vi "WPILogWaveformFromIndex.vi"(7 "XY Graph":refnum<vi>, 8 "error in (no error)":errorcluster, 9 "Index":i32, 10 "Graph Data":cluster{"X":dbl[], "Y":dbl[]}[](array[cluster]), 11 "Data Value Reference in":refnum<data-value>) -> (0 "error out":errorcluster, 2 "Graph Out":cluster{"X":dbl[], "Y":dbl[]}[](array[cluster]), 3 "Data Value Reference out":refnum<data-value>)   [LabVIEW 2020]
uses:
  Typedef/WPILibLog.ctl
  Typedef/Header.ctl
  Typedef/Entry.ctl
  Typedef/Record.ctl
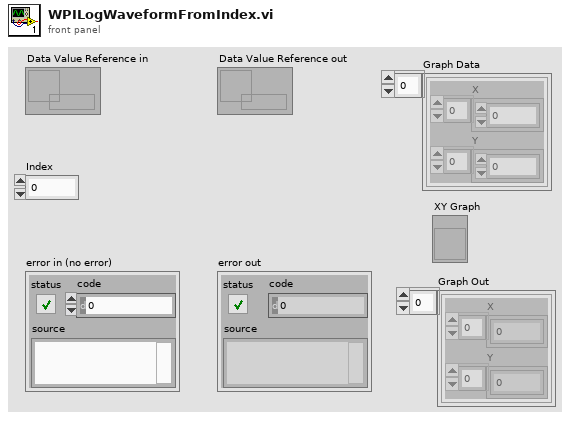
[diagram p1: front panel]
types:
  T1 = typedef "WPILibLog.ctl" = cluster{"Header":T2, "Record Start Idx":i32, "Entries":map{u32, T3}, "file ref":refnum<file>, "Finished Entries":T3[], "raw data":u8[]}
  T2 = typedef "Header.ctl" = cluster{"Header String":string, "Version":dbl, "Header Extra String Length":u32, "Header Extra String":string}
  T3 = typedef "Entry.ctl" = cluster{"ID":u32, "Records":T4[], "Finished?":bool, "Name":string, "Type":string, "Metadata":string, "RecordCnt":i32}
  T4 = typedef "Record.ctl" = cluster{"raw data":u8[], "ID":u32, "Size (bytes)":u32, "Timestamp":u64}
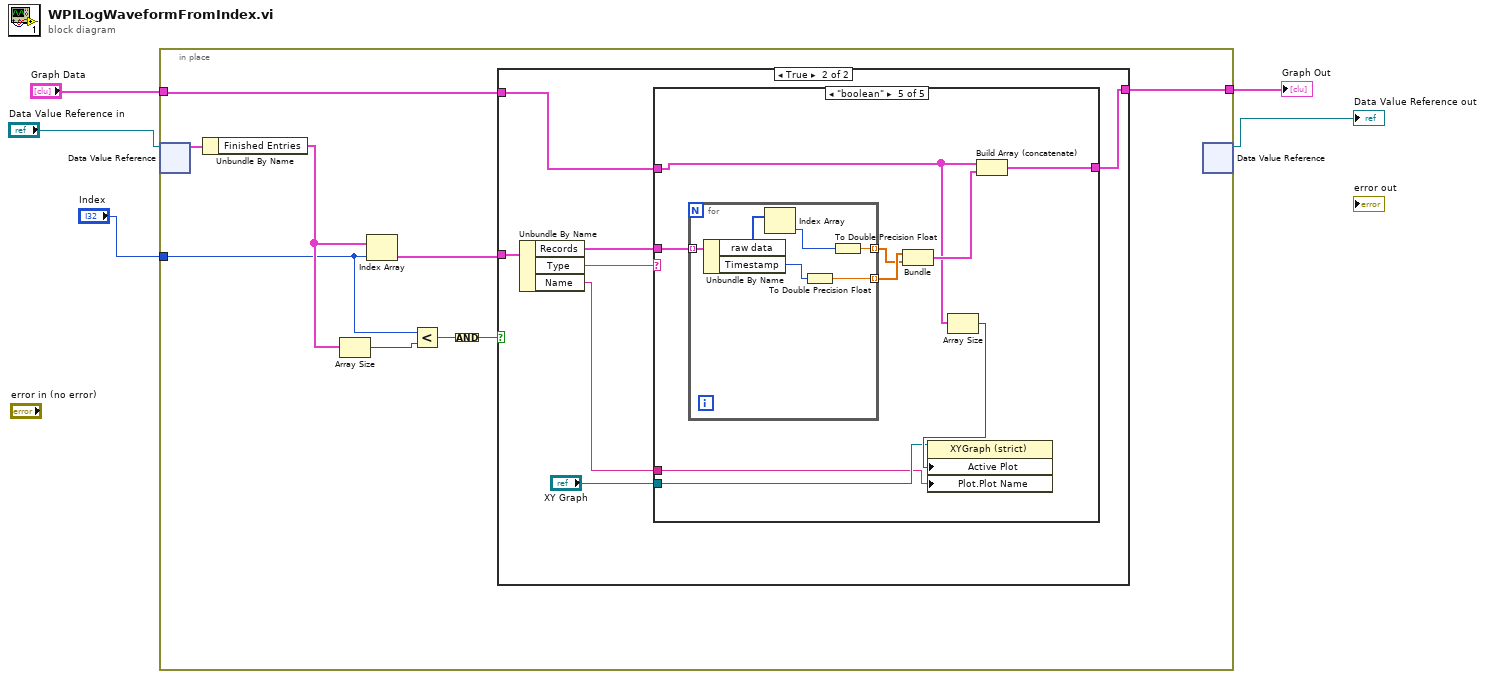
[diagram p0: block diagram]
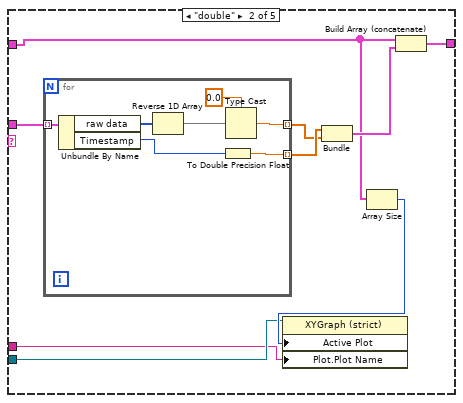
[diagram p4: hidden frame]
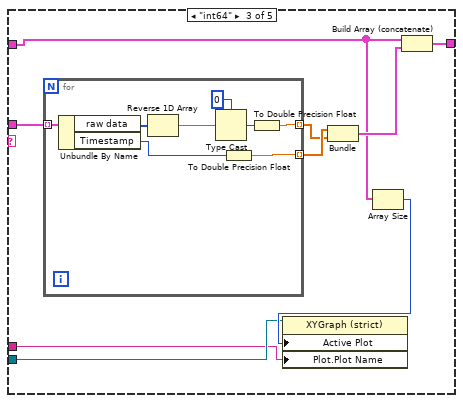
[diagram p5: hidden frame]
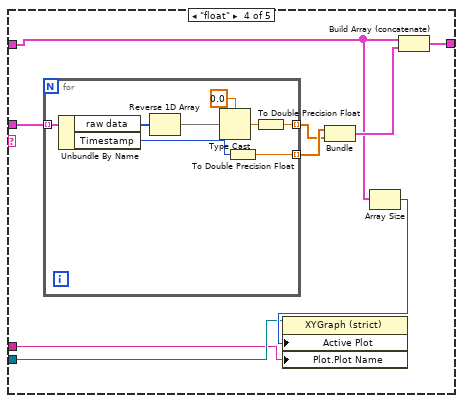
[diagram p6: hidden frame]
diagram:
  n1 = in-place {
    in-place-border: "Index" -> [w12]
    in-place-border: "Graph Data" -> [w7]
    in-place-border: [w6] -> w1
    n2 = in-place-dvr #1("Data Value Reference in") -> (w14:T1)  [unwired: 1 out]
    n3 = Unbundle By Name(w14) -> ("Finished Entries"=w13:T3[])
    n4 = Array Size(array=w13) -> (size(s)=w11:i32)
    n5 = Index Array(array=w13, index=w12) -> (element=w8:T3)
    n6 = Less?(x=w12, y=w11) -> (x < y?=w10:bool)
    n7 = Compound Arithmetic op=AND(w10) -> (w9:bool)
    n8 = case shown="True" w9 {
      tunnel: w8 -> [_ w22]
      tunnel: w7 -> [w15 w19]
      tunnel: [w15 w18] -> w6
      frame False {
      }
      frame True {
        n9 = Unbundle By Name(w22) -> ("Records"=w20:T4[], "Type"=w21:string, "Name"=w16:string)
        n10 = case shown="\"boolean\"" w21 {
          tunnel: w20 -> [_ w32 w48 w65 w82]
          tunnel: w19 -> [w23 w27 w43 w60 w77]
          tunnel: [w23 w28 w44 w61 w78] -> w18
          tunnel: "XY Graph" -> [_ w25 w41 w58 w75]
          tunnel: w16 -> [_ w24 w40 w57 w74]
          frame Default {
            # "Invalid Type, dont add"
          }
          frame "double" {
            n11 = for {
              tunnel: w32 -> [w39] mode=indexing
              tunnel: [w36] -> w30 mode=indexing
              tunnel: [w35] -> w31 mode=indexing
              n12 = Unbundle By Name(w39) -> ("raw data"=w38:u8[], "Timestamp"=w34:u64)
              n13 = Reverse 1D Array(array=w38) -> (reversed array=w33:u8[])
              n14 = To Double Precision Float(number=w34) -> (double precision float=w35:dbl)
              n15 = Type Cast(type=0.0, x=w33) -> (*(type *) &x=w36:dbl)
            }
            n16 = Bundle(w31, w30) -> (w29:cluster{dbl[], dbl[]})  [unwired: 1 in]
            n17 = Array Size(array=w27) -> (size(s)=w26:i32)
            n18 = property class="XYGraph (strict)"(reference=w25, "Active Plot"=w26, "Plot.Plot Name"=w24) -> ()  [unwired: 1 in, 2 out]
            n19 = Build Array (concatenate)(w27, w29) -> (w28:cluster{"X":dbl[], "Y":dbl[]}[])
          }
          frame "int64" {
            n20 = for {
              tunnel: w48 -> [w56] mode=indexing
              tunnel: [w51] -> w46 mode=indexing
              tunnel: [w52] -> w47 mode=indexing
              n21 = Unbundle By Name(w56) -> ("raw data"=w55:u8[], "Timestamp"=w50:u64)
              n22 = Reverse 1D Array(array=w55) -> (reversed array=w49:u8[])
              n23 = Type Cast(type=i64 0, x=w49) -> (*(type *) &x=w53:i64)
              n24 = To Double Precision Float(number=w50) -> (double precision float=w52:dbl)
              n25 = To Double Precision Float(number=w53) -> (double precision float=w51:dbl)
            }
            n26 = Bundle(w47, w46) -> (w45:cluster{dbl[], dbl[]})  [unwired: 1 in]
            n27 = Array Size(array=w43) -> (size(s)=w42:i32)
            n28 = property class="XYGraph (strict)"(reference=w41, "Active Plot"=w42, "Plot.Plot Name"=w40) -> ()  [unwired: 1 in, 2 out]
            n29 = Build Array (concatenate)(w43, w45) -> (w44:cluster{"X":dbl[], "Y":dbl[]}[])
          }
          frame "float" {
            n30 = for {
              tunnel: w65 -> [w73] mode=indexing
              tunnel: [w67] -> w63 mode=indexing
              tunnel: [w68] -> w64 mode=indexing
              n31 = Unbundle By Name(w73) -> ("raw data"=w72:u8[], "Timestamp"=w69:u64)
              n32 = Reverse 1D Array(array=w72) -> (reversed array=w66:u8[])
              n33 = Type Cast(type=sgl 0.0, x=w66) -> (*(type *) &x=w70:sgl)
              n34 = To Double Precision Float(number=w69) -> (double precision float=w68:dbl)
              n35 = To Double Precision Float(number=w70) -> (double precision float=w67:dbl)
            }
            n36 = Bundle(w64, w63) -> (w62:cluster{dbl[], dbl[]})  [unwired: 1 in]
            n37 = Array Size(array=w60) -> (size(s)=w59:i32)
            n38 = property class="XYGraph (strict)"(reference=w58, "Active Plot"=w59, "Plot.Plot Name"=w57) -> ()  [unwired: 1 in, 2 out]
            n39 = Build Array (concatenate)(w60, w62) -> (w61:cluster{"X":dbl[], "Y":dbl[]}[])
          }
          frame "boolean" {
            n40 = for {
              tunnel: w82 -> [w88] mode=indexing
              tunnel: [w85] -> w80 mode=indexing
              tunnel: [w86] -> w81 mode=indexing
              n41 = Unbundle By Name(w88) -> ("raw data"=w84:u8[], "Timestamp"=w87:u64)
              n42 = Index Array(array=w84) -> (element=w83:u8)  [unwired: 1 in]
              n43 = To Double Precision Float(number=w87) -> (double precision float=w86:dbl)
              n44 = To Double Precision Float(number=w83) -> (double precision float=w85:dbl)
            }
            n45 = Bundle(w81, w80) -> (w79:cluster{dbl[], dbl[]})  [unwired: 1 in]
            n46 = Array Size(array=w77) -> (size(s)=w76:i32)
            n47 = property class="XYGraph (strict)"(reference=w75, "Active Plot"=w76, "Plot.Plot Name"=w74) -> ()  [unwired: 1 in, 2 out]
            n48 = Build Array (concatenate)(w77, w79) -> (w78:cluster{"X":dbl[], "Y":dbl[]}[])
          }
        }
      }
    }
    n49 = in-place-dvr #1() -> (→"Data Value Reference out":refnum<data-value>)  [unwired: 1 in, 1 out]
  }
  "Graph Out" <- w1
